vi "Disconnect.vi"(8 "error in (no error)":errorcluster, 11 "midi in in":refnum<class "midi in.lvclass">) -> (0 "error out":errorcluster)   [LabVIEW 2020, in "midi in.lvclass"]
uses:
  midi in.lvclass
  midi in.lvclass/midi in.ctl
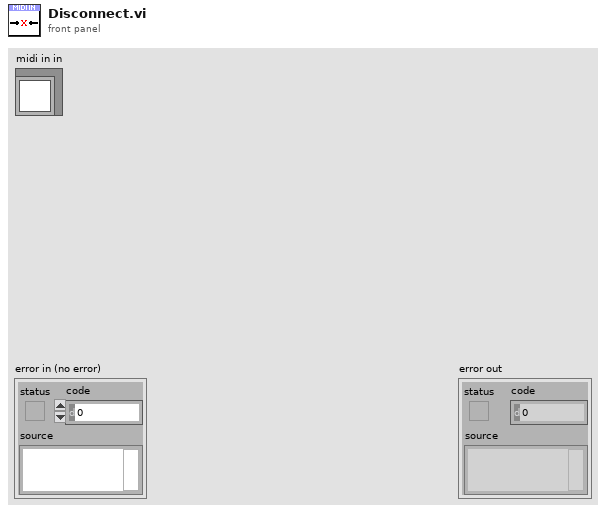
[diagram p1: front panel]
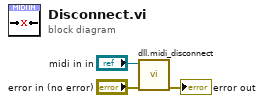
[diagram p0: block diagram]
diagram:
  n1 = call "dll.midi_disconnect.vi"("error in (no error)"="error in (no error)", "LabVIEW-MIDI-XPLAT in"="midi in in") -> ("error out"=→"error out":errorcluster)  [unwired: 8 in, 1 out]
